vi "Write Shutdown Timeout.vi"(8 "error in (no error)":errorcluster, 10 "Shutdown Timeout":u32, 11 "Watchdog in":refnum<class "Watchdog.lvclass">) -> (0 "error out":errorcluster, 3 "Watchdog out":refnum<class "Watchdog.lvclass">)   [LabVIEW 2017, in "Watchdog.lvclass"]
uses:
  <vilib>/NI/Software Watchdog/Watchdog/Watchdog.lvclass
  <vilib>/NI/Software Watchdog/Watchdog/Watchdog.lvclass/Watchdog.ctl
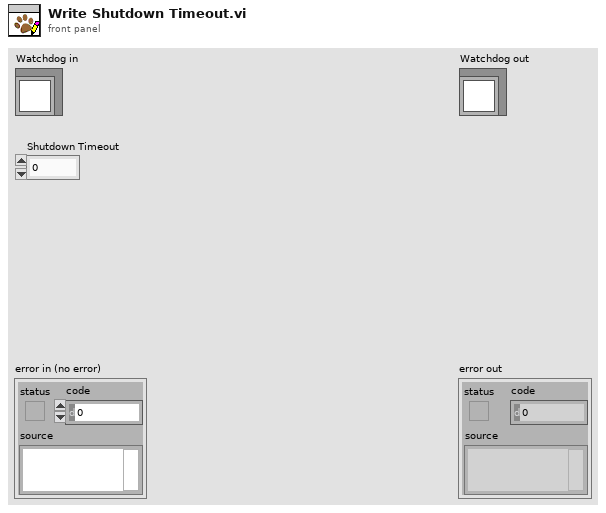
[diagram p1: front panel]
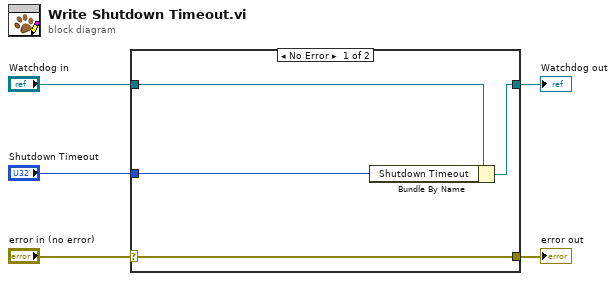
[diagram p0: block diagram]
diagram:
  n1 = case shown="No Error" "error in (no error)" {
    selector: "error in (no error)" -> [w9 w10]
    tunnel: [w9 w10] -> w4
    tunnel: [w7 w11] -> w2
    tunnel: "Watchdog in" -> [w8 w11]
    tunnel: "Shutdown Timeout" -> [w6 _]
    frame No Error {
      n2 = Bundle By Name(cluster=w8, "Shutdown Timeout"=w6) -> (w7:refnum<class "Watchdog.lvclass">)
    }
    frame Error {
    }
  }
  "error out" <- w4
  "Watchdog out" <- w2
